vi "HFRR ADV v025 new software.vi"() -> ()   [LabVIEW 2025] (continued)
  # "Calibrates the ambient air temperature sensor. \nUsed for environmental chamber monitoring."
  # "Set B\n60 °C\nHigh-point calibration"
  # "Set A\n0 °C\nIce-point calibration"
  # "Set B\n60 °C\nHigh-point calibration"
  # "Set A\n0 °C\nIce-point calibration"
  # "Select Temperature Sensor"
  # "Choose which temperature sensor you are calibrating. Both use the same two-\npoint procedure: 0 °C (ice-point) and 60 °C (high-point)."
  # "Step 1 — Reference Instrument Setup"
  # "Connect a calibrated reference to the DUT port. This calibration performs two sets: one at 0 °C and one at 60 °C."
  # "Set A\n0 °C\nIce-point calibration"
  # "Set B\n60 °C\nHigh-point calibration"
  # "Allow the temperature bath to stabilise for at least 2 minutes at each set-point before recording the reading."
  # "Step 2 — Set A:  0 °C Calibration"
  # "Connect the  0 °C reference connector. Wait for the temperature to stabilise. Once stable, and click Record Point."
  # "Step 3 — Set A:  60 °C Calibration"
  # "Connect the  60 °C reference connector. Wait for the temperature to stabilise. Once stable, and click Record Point."
  # "Step 1 — Reference Instrument Setup"
  # "Connect a calibrated reference to the DUT port. This calibration performs two sets: one at 0 °C and one at 60 °C."
  # "Set A\n0 °C\nIce-point calibration"
  # "Set B\n60 °C\nHigh-point calibration"
  # "Allow the temperature bath to stabilise for at least 2 minutes at each set-point before recording the reading."
  # "Step 2 — Set A:  0 °C Calibration"
  # "Connect the  0 °C reference connector. Wait for the temperature to stabilise. Once stable, and click Record Point."
  # "Step 3 — Set A:  60 °C Calibration"
  # "Connect the  60 °C reference connector. Wait for the temperature to stabilise. Once stable, and click Record Point."
  # "System Control Commands\nS;1 - Starts the full automation cycle (Runs Priming-humidify till 70RH sequence first, then switches to Maintenance).\nS;0 - Stops the system immediately and enters Standby mode (Safe State: All actuators OFF).\nM;1 - Skips the priming sequence and jumps directly to Maintenance mode (PID control).\nR;1 - Resets the logic state machine and clears all errors, returning to Standby.\nService Mode (Manual Control)\nX;1 - Enters Manual Service Mode. This disables all automatic logic, sensor safety checks, and timers.\nX;0 - Exits Manual Service Mode and returns to Standby (Safe State).\nActuator Commands (Only work after sending X;1)\nP;[0-255] - Sets the Pump PWM. Note that this is Active Low (0 = Max Flow, 255 = Pump OFF).\nF;I;[0-255] - Sets the Intake Fan speed (0 = OFF, 255 = Max Speed).\nF;O;[0-255] - Sets the Exhaust Fan speed (0 = OFF, 255 = Max Speed).\nD;1 - Turns the Dehumidifier Relay ON.\nD;0 - Turns the Dehumidifier Relay OFF."
  # "%RH"
  # "ISO : WS1.4"
  # "Start test and end test log--- done\nDisable heater ON and Humidity ON during the test --- done\ntemprature and ---done\nhumidity reach log\nauto start run true logic and log\nmanual start log once"
  # "Reference Fluid Information"
  # "Note:\nMake sure to place all images in the folder \"C:\\WinDucom\\im\" before clicking on \"Import Image.\""
  # "NOTE:\nPlace all the images in the path \"C:\\WinDucom\\im\" before clicking on Import Image"
  # "Wear Scar Measurements"
  # "Reference Fluid Information"
  # "Graph :"
types:
  T1 = enum32{"Home", "Dashboard", "Imaging", "Report", "Analysis", "About", "Test Setup", "Advance", "Calibration"}
  T2 = enum32{"HOME", "Test Setup", "Acquire", "Adv Scar", "Adv Scar Report", "Compare Files", "Calibration", "About", "Advance", "Mooha"}
  T3 = enum16{"ASTM D6079", "ISO 12156", "CEC F-096-A-06", "Custom"}
  T4 = enum32{"Dashboard 1", "Dashboard 2", "Dashboard 3"}
  T5 = enum32{"COF", "Friction", "ECR", "Temperature", "Humidity", "Stroke"}
  T6 = enum32{"Coefficient Of Friction", "Air Temperature", "Humidity", "Stroke", "Sample Temperature", "Electrical Contact Resistance", "Frequency", "Air Temp vs Rh"}
  T7 = enum32{"Main", "Stroke", "Friction", "Temperature"}
  T8 = enum32{"Stroke Calibration", "Friction Force Calibration", "Temperature Calibration"}
  T9 = enum32{"Step 1", "Step 2", "Step 3", "Step 4", "Step 5", "Step 6", "Step 7", "Step 8", "Step 9"}
  T10 = enum32{"Test Progress", "Stroke Points Completed"}
  T11 = enum32{"Main", "Step 1", "Step 2", "Step 3", "Air Step 1", "Air Step 2", "Air Step 3"}
  T12 = enum32{"COMMUNICATION", "CALIBRATION", "Temp Variables", "Camera", "WO 2465 (1)", "WO 2465 (2)", "WO 2465 (3)"}
  T13 = typedef "Auto Start enum.ctl" = enum16{"Init", "Humidity & Temperature On", "Reach point", "Maintain Stage", "Start Stage", "close", "Exit"}
  T14 = typedef "imagedata.ctl" = cluster{"image type":i32, "image depth":i32, "image":u8[], "mask":u8[], "colors":u32[], "Rectangle":cluster{"left":i16, "top":i16, "right":i16, "bottom":i16}}
  T15 = enum32{"HOME", "Test Setup", "Acquire", "Compare Files", "Print Report", "About", "Advance", "Mooha"}
  T16 = cluster{"Read Heave and Surge":string, "Bytes at Heave Port":dbl, "Heave and Surge COM Port:":refnum<visa-resource-name>, "Com Port 2":refnum<visa-resource-name>, "Residual Due":string, "Heave COM Status 2":bool, "Heave COM Status":bool, "Port 2":bool, "Sway PPR":dbl, "Surge PPR":dbl, "Heave PPR":dbl, "Sway Pitch":dbl, "Surge Pitch":dbl, "Heave Pitch":dbl, "Sway Pulses/mm":dbl, "Surge Pulses/mm":dbl, "Heave Pulses/mm":dbl, "inner loop":dbl, "Read Heave and Surge 2":string, "String 36":string, "Write S":bool, "WriteCC1":string[], "Heave COM Loop":i32, "LastCom":string, "EXIT":bool, "Error Heave":errorcluster}
  T17 = enum8{"Enabled", "Disabled", "Disabled and Grayed Out"}
  T18 = enum32{"HOME", "Test Setup", "Acquire", "Adv Scar", "Adv Scar Report", "Compare Files", "About", "Advance", "Mooha"}
  T19 = typedef "POST ANALYSIS ENUM.ctl" = enum16{"OPEN EXE", "INIT", "OPEN FILE", "FIT", "DRAW REC", "DRAW LINE", "PAN", "ZOOM IN", "ZOOM OUT", "SET ZOOM", "CLEAR ROI", "GET MEASUREMENTS", "RESIZE MODE", "STREAM START", "STREAM STOP", "SHOW UI", "MINIMIZE UI", "HIDE UI", "CKISE APP", "CLOSE CONNECTION", "SAVE IMAGE", "SET ROI COLOR", "READ", "TCP CHECK", "CLOSE"}
  T20 = typedef "CAMERA LIVE FEED ENUM.ctl" = enum16{"OPEN EXE", "INIT", "READ", "CAMERA CONNECT", "CAMERA START", "CAMERA STOP", "CAMERA GRAY", "CAMERA RGB", "CAMERA MINIMIZE", "CAMERA CLOSE", "CAMERA MODE LIST", "CAMERA MODE SET", "CAMERA RESTORE", "CAMERA SAVE", "CLOSE"}
  T21 = enum16{"Always On", "Always Off", "Off While Running"}
  T22 = enum32{"Home", "Dashboard", "Imaging", "Report", "Analysis", "About", "Test Setup", "Advance"}
  T23 = cluster{"File Name":string, "Test Method":string, "Operator":string, "Fuel Description":string, "Date and time":string}
  T24 = enum32{"Home", "Dashboard", "Imaging", "Report", "Analysis", "About", "Test Setup"}
  T25 = enum32{"HOME", "Test Setup", "Acquire", "Compare Files", "About", "Advance", "Mooha"}
  T26 = enum16{"deny read/write", "deny write-only", "deny none"}
  T27 = typedef "NI_ReportGenerationCore.lvlib/HTML Report Image Alignment.ctl" = enum16{"(default)", "LEFT", "RIGHT", "TOP", "TEXTTOP", "MIDDLE", "ABSMIDDLE", "BASELINE", "BOTTOM", "ABSBOTTOM"}
  T28 = enum16{"open", "replace", "create", "open or create", "replace or create", "replace or create with confirmation"}
  T29 = enum16{"INIT", "READ", "MANUAL WRITE", "WRITE", "CLOSE", "ERROR INIT"}
  T30 = enum16{"open", "open or create", "create or replace", "create", "open (read only)"}
  T31 = cluster{"Mode":enum16{"RTU", "ASCII"}, "Slave Address":u8}
diagram:
  w3 = 0.0 ("ch0_filt")
  w5 = -9999999.0 ("max_ch0")
  w6 = 9999999.0 ("min_ch0")
  w17 = FALSE ("Visible")
  w18 = T17."Enabled" ("Disabled")
  w21 = FALSE ("Visible")
  w20 = FALSE ("Humidity Off Command")
  w36 = "" ("USER ID")
  (unwired) T18."HOME" ("Main Tab")
  # "[CH1]    - FF\n[CH2]   - TEMPERATURE\n[CH3]    - Humidity\n[CH4]    - AIR TEMP\n[CH5]\\- Visa Uno\n[CH6] \\- Visa Due\n[CH7]  \\- file path\n[CH8]   - Displacement Gain\n[CHA]   - Stroke Gain\n[CHB]   - Stroke PID Gain\n[CHC]   -Language Selection\n[CHD]   -Power +\n[CHE]   -Power_\n[CHF]   -Heater\n[CHG]   -Humidity Wet\n[CHH]   -Humidity Dry\n[CHI]   -Integral Time \n[CHIJ   -Air intercept\n[CHI]   -Temp Intercept"
  n1 = local write "Cal Password"("" ("Cal Password")) -> ()
  n2 = property on="Auto Start Test" class="Bool (strict)"("Visible"=TRUE) -> ()  [unwired: 2 in, 2 out]
  n3 = property on="FRICVALZ 2" class="Bool (strict)"("DisabledEnum"=w18) -> ()  [unwired: 2 in, 2 out]
  n4 = property on="FRICVALZ 4" class="Bool (strict)"("DisabledEnum"=w18) -> ()  [unwired: 2 in, 2 out]
  n5 = property on="FRICVALZ 3" class="Bool (strict)"("DisabledEnum"=w18) -> ()  [unwired: 2 in, 2 out]
  n6 = property on="About" class="Clust (strict)"("Visible"=FALSE) -> ()  [unwired: 2 in, 2 out]
  n7 = property on="Wrong Password" class="Str"("Visible"=w17) -> ()  [unwired: 2 in, 2 out]
  n8 = property on="Calibration 2" class="TabCtl (strict)"("Visible"=w17) -> ()  [unwired: 2 in, 2 out]
  n9 = flat-sequence {
    tunnel: [w58] -> w2
    tunnel: [w103] -> w28
    tunnel: w2 -> [w98]
    tunnel: [w104] -> w30
    tunnel: w28 -> [w104]
    tunnel: w30 -> [w167]
    tunnel: [w167] -> w29
    tunnel: w29 -> [w198]
    tunnel: [w198] -> w39
    tunnel: w39 -> [w205]
    tunnel: [w211] -> w27
    tunnel: [w199] -> w26
    tunnel: [w253] -> w1
    tunnel: [w252] -> _
    tunnel: w27 -> [w252]
    tunnel: w26 -> [w253]
    frame #0 {
      n10 = call "CLOSE CONNECTION.vi"("error in (no error)"="error in (no error) 2") -> ("error out"=w63:errorcluster)  [unwired: 10 in]
      n11 = call <vilib>:"Clear Errors.vi"("error in (no error)"=w63) -> ("error out"=w62:errorcluster)  [unwired: 5 in, 1 out]
      n12 = disable-structure shown="Enabled" {
        disable-tunnel: w62 -> [w90 _]
        disable-tunnel: [w89 _] -> w61
        frame Enabled {
          n13 = call <userlib>:"Fit VI window to Largest Dec.vi"("error in (no error)"=w90, "border spacing (2 px)"=1) -> ("error out"=w93:errorcluster, "dup VI Ref"=w97:refnum<vi>)  [unwired: 4 in]
          n14 = invoke on="Invoke Node" class="VI" method="FP.Run-Time Position.Maximized"(reference=w97, error in=w93) -> (error out=w94:errorcluster)  [unwired: 2 in, 3 out]
          n15 = call <vilib>:"Clear Errors.vi"("error in (no error)"=w94) -> ("error out"=w96:errorcluster)  [unwired: 5 in, 1 out]
          n16 = control-ref of="This VI"() -> (w88:refnum<vi>)
          n17 = invoke on="Invoke Node" class="VI" method="Default Vals.Reinit All"(reference=w88, error in=w96) -> (reference out=w92:refnum<vi>, error out=w91:errorcluster)  [unwired: 1 in, 1 out]
          n18 = Close Reference(reference=w92, error in (no error)=w91) -> (error out=w89:errorcluster)
        }
        frame Disabled {
        }
      }
      n19 = call "Stall Data Flow.vim"("value in"=w61, "milliseconds to wait"=u32 2000) -> ("value out"=w60:errorcluster)  [unwired: 1 out]
      n20 = call "Read Config.vi"("error in (no error)"=w60) -> ("error out"=w58:errorcluster, "STROKE PARAMETERS"=w69:dbl[], "ADC PARAMETERS"=w70:dbl[], "PID  PARAMETERS"=w71:dbl[], "Stroke Calibration"=w68:string)  [unwired: 6 in]
      n21 = Index Array(array=w69) -> (element #1=w86:dbl, element #2=w87:dbl)  [unwired: 2 in]
      n22 = Index Array(array=w70) -> (element #1=w82:dbl, element #2=w83:dbl, element #3=w84:dbl, element #4=w85:dbl)  [unwired: 4 in]
      n23 = Index Array(array=w71) -> (element #1=w73:dbl, element #2=w74:dbl, element #3=w75:dbl, element #4=w76:dbl, element #5=w77:dbl, element #6=w78:dbl, element #7=w79:dbl, element #8=w80:dbl, element #9=w81:dbl)  [unwired: 9 in]
      n24 = local write "milliseconds to wait"(w73) -> ()
      n25 = local write "dt"(w74) -> ()
      n26 = local write "kp"(w75) -> ()
      n27 = local write "ki"(w76) -> ()
      n28 = local write "kd"(w77) -> ()
      n29 = local write "max_step_change"(w78) -> ()
      n30 = local write "max_amplitude"(w79) -> ()
      n31 = local write "min_amplitude"(w80) -> ()
      n32 = local write "startup_cmd"(w81) -> ()
      n33 = local write "VREF"(w82) -> ()
      n34 = local write "ADC_Resolution"(w83) -> ()
      n35 = local write "PIEZO_CAL_FACTOR"(w84) -> ()
      n36 = local write "NORMAL_FORCE"(w85) -> ()
      n37 = local write "STROKE FILTER"(w86) -> ()
      n38 = local write "Add up Stroke"(w87) -> ()
      n39 = Spreadsheet String To Array(delimiter (Tab)=";", format string="", spreadsheet string=w68, array type (2D Dbl)=dbl[] []) -> (array=w72:dbl[])
      n40 = local write "calibration values"(w72) -> ()
    }
    frame #1 {
      n41 = property on="Auto Scar Check" class="Clust (strict)"("Visible"=TRUE) -> ()  [unwired: 2 in, 2 out]
      n42 = property on="Sign In" class="Bool (strict)"("DisabledEnum"=T17."Disabled" ("Disabled")) -> ()  [unwired: 2 in, 2 out]
      n43 = local write "sign in temp"(FALSE ("sign in temp")) -> ()
      n44 = call "dialog box.vi"("Status"="Before starting the test, verify that the microscope cable is connected.", "error in"=w98) -> ("error out"=w103:errorcluster)  [unwired: 8 in]
    }
    frame #2 {
      (unwired) TRUE ("Re-Initialise")
      w110 = FALSE ("Upld AR 2")
      # "kkkkk"
      # "C:\\Windows\\wndcm_pw_stdED hfrr.txt"
      # "C:\\LAB-IQ NXT"
      # "C:\\LAB-IQ NXT\\wndcm_pw_stdED hfrr.txt"
      # "password file"
      n45 = Current VI's Path() -> (path=w123:path)
      n46 = Strip Path(path=w123) -> (stripped path=w116:path)  [unwired: 1 out]
      n47 = local write "Json End Flg"(w110) -> ()
      n48 = local write "Json St Flg"(w110) -> ()
      n49 = local write "main tab sub"(enum32{"Page 1", "Page 2"}."Page 1" ("main tab sub")) -> ()
      n50 = local write "Main Tab Display"(T4."Dashboard 1" ("Main Tab Display")) -> ()
      n51 = local write "Main Tab"(T2."HOME" ("Main Tab")) -> ()
      n52 = Path To String(path=w116) -> (string=w118:string)
      n53 = Search/Split String(string=w118, search string/char (-)=".exe") -> (match + rest of string=w120:string)  [unwired: 1 in, 2 out]
      n54 = Match True/False String(2:".vi" ("false string"), 3:".exe" ("true string"), 4:w120) -> (0:w117:bool)  [unwired: 1 out]
      n55 = List Folder(path=path "C:/LAB-IQ" ("directory path"), pattern="*.txt") -> (filenames=w129:string[])  [unwired: 2 in, 3 out]
      n56 = case shown="True" w117 {
        tunnel: w116 -> [w138 w140]
        tunnel: [w138 w139] -> w114
        frame False {
        }
        frame True {
          n57 = Strip Path(path=w140) -> (stripped path=w139:path)  [unwired: 1 out]
        }
      }
      n58 = Search 1D Array(1D array=w129, element="wndcm_pw_stdED hfrr.txt") -> (index of element=w132:i32)  [unwired: 1 in]
      n59 = Equal?(x=w132, y=-1) -> (x = y?=w127:bool)
      n60 = Path To String(path=w114) -> (string=→"Gain path":string)
      n61 = case shown="True" w127 {
        frame False {
        }
        frame True {
          n62 = String To Byte Array(string="123\n") -> (unsigned byte array=w145:u8[])
          n63 = Array Size(array=w145) -> (size(s)=w144:i32)
          n64 = for {
            N: w144 -> [_]
            tunnel: w145 -> [w158]
            tunnel: [w155] -> w147 mode=indexing
            tunnel: w144 -> [w150]
            i -> [w148]
            n65 = Decrement(x=w150) -> (x-1=w151:i32)
            n66 = Index Array(array=w158, index=w148) -> (element=w157:u8)
            n67 = Equal?(x=w148, y=w151) -> (x = y?=w152:bool)
            n68 = Number To Decimal String(number=w157) -> (decimal integer string=w156:string)  [unwired: 1 in]
            n69 = Select(t="", s=w152, f="\r") -> (s? t:f=w149:string)
            n70 = Concatenate Strings(w156, w149) -> (w155:string)
          }
          n71 = local read "file path"() -> (w141:path)
          n72 = Concatenate Strings(w147) -> (w143:string)
          n73 = call <vilib>:"Write Characters To File.vi"("append to file? (new file:F)"=FALSE, "character string"=w143, "file path (dialog if empty)"=w141) -> ()  [unwired: 2 in, 1 out]
        }
      }
      n74 = local write "FLAG 2"(0.0 ("FLAG 2")) -> ()
      n75 = local write "conststatus"(0.0 ("rpm value : 2")) -> ()
      n76 = local write "EVENT LOG"("") -> ()
      n77 = local write "COUNT"(0 ("COUNT")) -> ()
      n78 = local write "clk"(0.0 ("clk")) -> ()
      n79 = local write "Flag"(0.0 ("Flag")) -> ()
      n80 = local write "Lan flag"(0.0 ("Lan flag")) -> ()
      n81 = local write "Com flag"(u32 0 ("Com flag")) -> ()
      n82 = local write "refresh flag"(FALSE ("refresh flag")) -> ()
      n83 = local write "Upld AR 2"(TRUE ("Upld AR 2")) -> ()
      "file path" <- path "C:/LAB-IQ/wndcm_pw_stdED hfrr.txt" ("file path")
      "FF buffer" <- dbl[] [] ("FF buffer")
    }
    frame #3 {
      # "C:\\WinDucom\\calibrate WO 2391.dcf"
      n84 = String To Path(string="C:\\LAB-IQ\\Image Calibrate v01.dcf") -> (path=w162:path)
      n85 = String To Path(string="C:\\LAB-IQ\\calibrate WO 2465.dcf") -> (path=w166:path)
      n86 = Open/Create/Replace File "Open File"(file path (use dialog)=w166) -> (refnum out=w165:refnum<file>)  [unwired: 5 in, 2 out]
      n87 = Open/Create/Replace File ("Open File")(file path (use dialog)=w162) -> (refnum out=w161:refnum<file>)  [unwired: 5 in, 2 out]
      n88 = for {
        N: 4 -> [_]
        tunnel: w161 -> [w173]
        i -> [w169]
        n89 = Read from Text File ("Read File")(file (use dialog)=w173) -> (text=w174:string)  [unwired: 3 in, 3 out]
        n90 = String Subset(string=w174, offset (0)=6, length (rest)=10 ("length (rest)")) -> (substring=w170:string)
        n91 = Fract/Exp String To Number(string=w170) -> (number=w168:dbl)  [unwired: 3 in, 1 out]
        n92 = case shown="3" w169 {
          tunnel: w168 -> [w175 w176 _ w177 _]
          frame 0 {
            n93 = local write "5x Gain"(w175) -> ()
          }
          frame 1 {
            n94 = local write "10x Gain"(w176) -> ()
          }
          frame 2 {
          }
          frame 3 {
            n95 = local write "100x gain"(w177) -> ()
          }
          frame 4, Default {
          }
        }
      }
      n96 = for {
        N: 24 -> [_]
        tunnel: w165 -> [w186]
        i -> [w180]
        (unwired) TRUE ("line mode (F)")
        n97 = Read from Text File "Read File"(file (use dialog)=w186) -> (text=w185:string)  [unwired: 3 in, 3 out]
        n98 = Match Pattern(string=w185, regular expression="]") -> (after substring=w183:string)  [unwired: 1 in, 3 out]
        n99 = String Subset(string=w185, offset (0)=5, length (rest)=10 ("length (rest)")) -> (substring=w178:string)
        n100 = Fract/Exp String To Number(string=w178) -> (number=w179:dbl)  [unwired: 3 in, 1 out]
        n101 = Match Pattern(string=w183, regular expression="-") -> (before substring=w181:string)  [unwired: 1 in, 3 out]
        n102 = case shown="18" w180 {
          tunnel: w179 -> [_ _ _ _ _ _ _ _ _ _ w193 _ _ _ _ _ _ _ _ _ _ _ _ _ _]
          tunnel: w181 -> [_ _ _ _ w189 w190 w191 _ _ _ _ _ _ _ _ _ _ _ _ _ w194 _ w195 w196 _]
          frame 0 {
          }
          frame 1 {
          }
          frame 2 {
          }
          frame 3 {
          }
          frame 4 {
            n103 = local write "Com Port 1"(w189) -> ()
          }
          frame 5 {
            n104 = local write "Com Port 2"(w190) -> ()
            n105 = local write "visa due"(w190) -> ()
          }
          frame 6 {
            n106 = String To Path(string=w191) -> (path=w192:path)
            n107 = local write "File Path"(w192) -> ()
          }
          frame 7 {
          }
          frame 8 {
          }
          frame 9 {
          }
          frame 10 {
            n108 = local write "Language Selection"(w193) -> ()
          }
          frame 11 {
          }
          frame 12 {
          }
          frame 13 {
          }
          frame 14 {
          }
          frame 15 {
          }
          frame 16 {
          }
          frame 17 {
          }
          frame 18 {
          }
          frame 21 {
          }
          frame 22 {
            n109 = local write "Com Port 3"(w194) -> ()
          }
          frame 23 {
          }
          frame 19 {
            n110 = local write "C3 :"(w195) -> ()
          }
          frame 20 {
            n111 = local write "Camera Port :"(w196) -> ()
          }
          frame 24, Default {
          }
        }
      }
    }
    frame #4 {
      n112 = Wait (ms)(milliseconds to wait=u32 1000) -> ()  [unwired: 1 out]
    }
    frame #5 {
      w214 = u32 2000 ("milliseconds to wait")
      w241 = u32 2000 ("milliseconds to wait")
      n113 = call "CAMERA LIVE FEED FGV.vi"("Enum - Menu"=CAMERA_LIVE_FEED_ENUM."OPEN EXE", "error in (no error)"=w205) -> ("error out"=w247:errorcluster)  [unwired: 8 in, 1 out]
      n114 = call "IMAGE ANALYSIS.vi"("Enum"=POST_ANALYSIS_ENUM."OPEN EXE", "error in"=w205) -> ("error out"=w202:errorcluster)  [unwired: 8 in, 1 out]
      n115 = call "Stall Data Flow.vim"("value in"=w247, "milliseconds to wait"=w241) -> ("value out"=w245:errorcluster)  [unwired: 1 out]
      n116 = call "Stall Data Flow.vim"("value in"=w202, "milliseconds to wait"=u32 8000) -> ("value out"=w201:errorcluster)  [unwired: 1 out]
      n117 = call "CAMERA LIVE FEED FGV.vi"("Enum - Menu"=CAMERA_LIVE_FEED_ENUM."INIT", "error in (no error)"=w245) -> ("error out"=w243:errorcluster)  [unwired: 8 in, 1 out]
      n118 = call "IMAGE ANALYSIS.vi"("Enum"=POST_ANALYSIS_ENUM."INIT", "error in"=w201) -> ("error out"=w199:errorcluster)  [unwired: 8 in, 1 out]
      n119 = case shown="Error .." w243 {
        selector: w243 -> [w248 _]
        tunnel: [w248 _] -> w242
        frame No Error {
        }
        frame Error {
          n120 = One Button Dialog(message="Camera initialization error.\nPlease Restart the software") -> ()  [unwired: 1 in, 1 out]
        }
      }
      n121 = property on="Camera Port :" class="CmbBox"() -> ("Strings[]"=w239:string[], "Value"=w240:string)  [unwired: 2 in, 2 out]
      n122 = Search 1D Array(1D array=w239, element=w240) -> (index of element=w238:i32)  [unwired: 1 in]
      n123 = Type Cast(type=30, x=w238) -> (*(type *) &x=w236:i32)
      n124 = call "Stall Data Flow.vim"("value in"=w242, "milliseconds to wait"=w241) -> ("value out"=w218:errorcluster)  [unwired: 1 out]
      n125 = Add(x=w236, y=48) -> (x+y=w217:i32)
      n126 = call "CAMERA LIVE FEED FGV.vi"("Enum - Menu"=CAMERA_LIVE_FEED_ENUM."CAMERA CONNECT", "error in (no error)"=w218, "CAMERA PORT"=w217) -> ("error out"=w227:errorcluster)  [unwired: 7 in, 1 out]
      n127 = call "Stall Data Flow.vim"("value in"=w227, "milliseconds to wait"=u32 5000) -> ("value out"=w228:errorcluster)  [unwired: 1 out]
      n128 = call "CAMERA LIVE FEED FGV.vi"("Enum - Menu"=CAMERA_LIVE_FEED_ENUM."CAMERA MODE LIST", "error in (no error)"=w228) -> ("error out"=w230:errorcluster)  [unwired: 8 in, 1 out]
      n129 = call "Stall Data Flow.vim"("value in"=w230, "milliseconds to wait"=w214) -> ("value out"=w229:errorcluster)  [unwired: 1 out]
      n130 = call "CAMERA LIVE FEED FGV.vi"("Enum - Menu"=CAMERA_LIVE_FEED_ENUM."READ", "error in (no error)"=w229) -> ("error out"=w216:errorcluster, "data out"=→"Camera List":string)  [unwired: 8 in]
      n131 = Type Cast(type=30, x=0) -> (*(type *) &x=w210:i32)
      n132 = call "Stall Data Flow.vim"("value in"=w216, "milliseconds to wait"=w214) -> ("value out"=w215:errorcluster)  [unwired: 1 out]
      n133 = Add(x=w210, y=48) -> (x+y=w208:i32)
      n134 = call "CAMERA LIVE FEED FGV.vi"("Enum - Menu"=CAMERA_LIVE_FEED_ENUM."CAMERA MODE SET", "error in (no error)"=w215, "CAMERA MODE"=w208) -> ("error out"=w212:errorcluster)  [unwired: 7 in, 1 out]
      n135 = call "Stall Data Flow.vim"("value in"=w212, "milliseconds to wait"=u32 2000) -> ("value out"=w232:errorcluster)  [unwired: 1 out]
      n136 = call "CAMERA LIVE FEED FGV.vi"("Enum - Menu"=CAMERA_LIVE_FEED_ENUM."CAMERA START", "error in (no error)"=w232) -> ("error out"=w233:errorcluster)  [unwired: 8 in, 1 out]
      n137 = call "Stall Data Flow.vim"("value in"=w233, "milliseconds to wait"=u32 1000) -> ("value out"=w234:errorcluster)  [unwired: 1 out]
      n138 = call "CAMERA LIVE FEED FGV.vi"("Enum - Menu"=CAMERA_LIVE_FEED_ENUM."CAMERA MINIMIZE", "error in (no error)"=w234) -> ("error out"=w211:errorcluster)  [unwired: 8 in, 1 out]
    }
    frame #6 {
      n139 = case shown="No Error" w252 {
        frame No Error {
          n140 = property on="Auto Scar Check" class="Clust (strict)"("Visible"=FALSE) -> ()  [unwired: 2 in, 2 out]
        }
        frame Error {
        }
      }
      n141 = property on="Sign In" class="Bool (strict)"("DisabledEnum"=T17."Enabled" ("Disabled")) -> ()  [unwired: 2 in, 2 out]
      n142 = local write "sign in temp"(TRUE ("sign in temp")) -> ()
    }
  }
  n143 = local write "SCAR MEASURMENT"(enum32{"Auto Scar", "Manual Scar"}."Manual Scar" ("SCAR MEASURMENT")) -> ()
  n144 = local write "Temperature Off Command"(w20) -> ()
  n145 = local write "Main Dashboard Buttons"(T1."Home" ("Main Dashboard Buttons")) -> ()
  n146 = local write "Humidity Off Command"(w20) -> ()
  n147 = local write "CAMERA ROI MIN TEMP"(w20) -> ()
  n148 = local write "TEST FILE NAM,E SAVED"(w20) -> ()
  n149 = local write "LIVE FEED MIN TEMP"(w20) -> ()
  n150 = local write "SCAR MEASURMENT"(enum32{"Auto Scar", "Manual Scar"}."Manual Scar" ("SCAR MEASURMENT")) -> ()
  n151 = local write "Auto stop temp"(w21) -> ()
  n152 = local write "main tab sub"(enum32{"Page 1", "Page 2"}."Page 1" ("main tab sub")) -> ()
  n153 = local write "USERNAME"(w36) -> ()
  n154 = local write "Main Tab"(T2."HOME" ("Main Tab")) -> ()
  n155 = local write "USER ID"(w36) -> ()
  n156 = property on="Auto Scar Check  2" class="Clust (strict)"("Visible"=w21) -> (error out=w24:errorcluster)  [unwired: 2 in, 1 out]
  n157 = property on="Quit" class="Bool (strict)"("Value"=FALSE ("Quit")) -> (error out=w38:errorcluster)  [unwired: 2 in, 1 out]
  n158 = while {
    stop <- w255 stop-if-true
    n159 = event shown="[12] \"Cal Password\": Value Change" {
      selector: _ -> [_ _ _ _ _ _ _ _ _ _ _ _ _ _ _ _ _ _ _ _ _ _ _ _ _ _ _ _ _ _ _ _ _ _ _ _ _ _ _]
      dyn-events: _ -> [_ _ _ _ _ _ _ _ _ _ _ _ _ _ _ _ _ _ _ _ _ _ _ _ _ _ _ _ _ _ _ _ _ _ _ _ _ _ _]
      timeout: 100 -> [_ _ _ _ _ _ _ _ _ _ _ _ _ _ _ _ _ _ _ _ _ _ _ _ _ _ _ _ _ _ _ _ _ _ _ _ _ _ _]
      tunnel: [FALSE FALSE _ FALSE _ _ _ _ _ _ _ _ _ _ _ _ _ _ _ _ _ _ _ _ _ _ _ _ _ _ _ _ _ _ _ _ _ _ TRUE] -> w255
      event Timeout {
        n160 = event-data() -> ()  [unwired: 1 in, 3 out]
        n161 = disable-structure shown="Disabled" {
          frame Disabled {
            n162 = local read "Auto Start Test"() -> (w269:bool)
            n163 = local read "RUN"() -> (w270:bool)
            n164 = Or(x=w270, y=w269) -> (x .or. y?=w268:bool)
            n165 = case shown="True" w268 {
              frame False {
                w271 = TRUE ("PAUSE")
                n166 = call "ELAPSED TIMER VI - abort test.vi"("RESET"=w271, "PAUSE"=w271) -> ()  [unwired: 7 in, 3 out]
              }
              frame True {
                n167 = local read "Stroke 2"() -> (w276:dbl)
                n168 = local read "FF 3"() -> (w278:dbl)
                n169 = Equal?(x=w276, y=0.95 ("Stroke 2")) -> (x = y?=w273:bool)
                n170 = Equal?(x=w278, y=0.0 ("FF 3")) -> (x = y?=w274:bool)
                n171 = Or(x=w274, y=w273) -> (x .or. y?=w272:bool)
                n172 = case shown="True" w272 {
                  selector: w272 -> [_ w283]
                  frame False {
                    w279 = TRUE ("PAUSE")
                    n173 = call "ELAPSED TIMER VI - abort test.vi"("RESET"=w279, "PAUSE"=w279) -> ()  [unwired: 7 in, 3 out]
                  }
                  frame True {
                    n174 = Not(x=w283) -> (.not. x?=w282:bool)
                    n175 = call "ELAPSED TIMER VI - abort test.vi"("TARGET"=60.0, "RESET"=w282, "PAUSE"=FALSE) -> ("ELAPSED INDICATION"=w280:bool)  [unwired: 6 in, 2 out]
                    n176 = case shown="True" w280 {
                      frame False {
                      }
                      frame True {
                        n177 = stacked-sequence {
                          frame #0 {
                            w285 = FALSE
                            n178 = local write "RUN"(w285) -> ()
                            n179 = local write "Auto Start Test"(w285) -> ()
                          }
                          frame #1 {
                            n180 = One Button Dialog(message="Test stopped due to a communication error. Reconnect the C1 and C2 cables.") -> ()  [unwired: 1 in, 1 out]
                          }
                        }
                      }
                    }
                  }
                }
              }
            }
          }
          frame Enabled {
          }
        }
        n181 = Get Date/Time In Seconds() -> (seconds since 1Jan1904=w266:timestamp)
        n182 = Format Into String(format string="%<%I:%M:%S:%p %d:%B:%Y>T", w266) -> (resulting string=→"Time Stamp":string)  [unwired: 2 in, 1 out]
        n183 = local read "Service Password enable"() -> (w258:bool)
        n184 = local read "FILE"() -> (w263:string)
        n185 = call <vilib>:"Trim Whitespace.vi"("string"=w263) -> ("trimmed string"=w262:string)  [unwired: 1 in]
        n186 = String Length(string=w262) -> (length=w261:i32)
        n187 = Greater?(x=w261, y=1) -> (0:w259:bool)
        n188 = case shown="False" w259 {
          tunnel: w258 -> [w287 _]
          frame False {
            n189 = case shown="False" w287 {
              frame True {
                w288 = "Test Start In Service Mode" ("Tip Strip")
                w289 = T17."Enabled" ("Disabled")
                n190 = property on="Auto Start Test" class="Bool (strict)"("DisabledEnum"=w289, "TipStrip"=w288) -> ()  [unwired: 2 in, 2 out]
                n191 = property on="RUN" class="Bool (strict)"("DisabledEnum"=w289, "TipStrip"=w288) -> ()  [unwired: 2 in, 2 out]
              }
              frame False {
                w290 = "Enter File Name to Start Test" ("Tip Strip")
                w291 = T17."Disabled and Grayed Out" ("Disabled")
                n192 = property on="Auto Start Test" class="Bool (strict)"("DisabledEnum"=w291, "TipStrip"=w290) -> ()  [unwired: 2 in, 2 out]
                n193 = property on="RUN" class="Bool (strict)"("DisabledEnum"=w291, "TipStrip"=w290) -> ()  [unwired: 2 in, 2 out]
              }
            }
          }
          frame True {
            w292 = "" ("Tip Strip")
            w293 = T17."Enabled" ("Disabled")
            n194 = property on="Auto Start Test" class="Bool (strict)"("DisabledEnum"=w293, "TipStrip"=w292) -> ()  [unwired: 2 in, 2 out]
            n195 = property on="RUN" class="Bool (strict)"("DisabledEnum"=w293, "TipStrip"=w292) -> ()  [unwired: 2 in, 2 out]
          }
        }
      }
      event "RUN": Value Change {
        n196 = event-data() -> ()  [unwired: 1 in, 6 out]
        n197 = local read "RUN"() -> (w295:bool)
        n198 = case shown="False" w295 {
          frame False {
            n199 = flat-sequence {
              frame #0 {
                n200 = local write "START TEMP"(FALSE ("START TEMP")) -> ()
              }
              frame #1 {
                n201 = Wait (ms)(milliseconds to wait=u32 1500) -> ()  [unwired: 1 out]
              }
              frame #2 {
              }
              frame #3 {
                n202 = local write "Due Write"("VC;0") -> ()
              }
              frame #4 {
                n203 = Wait (ms)(milliseconds to wait=u32 1500) -> ()  [unwired: 1 out]
              }
              frame #5 {
                w304 = T17."Enabled" ("Disabled")
                (unwired) T22."Imaging" ("Main Dashboard Buttons")
                (unwired) T18."Adv Scar" ("Main Tab")
                w306 = "" ("FILE")
                n204 = local write "measured_stroke"(0.0 ("measured_stroke")) -> ()
                n205 = local write "Due Write"("VC;0") -> ()
                n206 = local write "FILE"(w306) -> ()
                n207 = local write "Batch Ref Num :"(w306) -> ()
                n208 = local write "Fuel Discription :"(w306) -> ()
                n209 = local write "Main Tab"(T2."Adv Scar" ("Main Tab")) -> ()
                n210 = local write "Remarks :"(w306) -> ()
                n211 = local write "Main Dashboard Buttons"(T1."Imaging" ("Main Dashboard Buttons")) -> ()
                n212 = local write "TEST FILE NAM,E SAVED"(FALSE ("TEST FILE NAM,E SAVED")) -> ()
                n213 = property on="Stroke ( mm )" class="WFChart (strict)"("History Data"=cluster{"y":dbl, dbl, "y":dbl}[] []) -> ()  [unwired: 2 in, 2 out]
                n214 = property on="Auto Start Test" class="Bool (strict)"("Visible"=TRUE) -> ()  [unwired: 2 in, 2 out]
                n215 = property on="FRICVALZ 2" class="Bool (strict)"("DisabledEnum"=w304) -> ()  [unwired: 2 in, 2 out]
                n216 = property on="FRICVALZ 4" class="Bool (strict)"("DisabledEnum"=w304) -> ()  [unwired: 2 in, 2 out]
                n217 = property on="FRICVALZ 3" class="Bool (strict)"("DisabledEnum"=w304) -> ()  [unwired: 2 in, 2 out]
              }
            }
          }
          frame True {
            n218 = flat-sequence {
              frame #0 {
                n219 = local write "Due Write"("VC;1") -> ()
              }
              frame #1 {
                n220 = Wait (ms)(milliseconds to wait=u32 2000) -> ()  [unwired: 1 out]
              }
              frame #2 {
                n221 = local write "Due Write"("VC;1") -> ()
              }
              frame #3 {
                n222 = Wait (ms)(milliseconds to wait=u32 2000) -> ()  [unwired: 1 out]
              }
              frame #4 {
                w314 = T17."Disabled" ("Disabled")
                n223 = property on="Auto Start Test" class="Bool (strict)"("Visible"=FALSE) -> ()  [unwired: 2 in, 2 out]
                n224 = local write "START TEMP"(TRUE ("START TEMP")) -> ()
                n225 = property on="FRICVALZ 2" class="Bool (strict)"("DisabledEnum"=w314) -> ()  [unwired: 2 in, 2 out]
                n226 = property on="FRICVALZ 4" class="Bool (strict)"("DisabledEnum"=w314) -> ()  [unwired: 2 in, 2 out]
                n227 = property on="FRICVALZ 3" class="Bool (strict)"("DisabledEnum"=w314) -> ()  [unwired: 2 in, 2 out]
              }
            }
          }
        }
      }
      event "Auto": Value Change {
        n228 = event-data() -> ()  [unwired: 1 in, 6 out]
        n229 = stacked-sequence {
          frame #0 {
            n230 = local write "FILE"("") -> ()
          }
          frame #1 {
            n231 = Get Date/Time In Seconds() -> (seconds since 1Jan1904=w320:timestamp)
            n232 = Format Into String(format string="%<%I_%M_%S_%p_%d_%B_%Y>T", w320) -> (resulting string=w319:string)  [unwired: 2 in, 1 out]
            n233 = local write "FILE"(w319) -> ()
          }
        }
        n234 = local read "Auto"() -> (w317:bool)
        n235 = Not(x=w317) -> (.not. x?=w316:bool)
        n236 = local write "Auto"(w316) -> ()
      }
      event "Auto Start Temp": Value Change {
        n237 = event-data() -> ()  [unwired: 1 in, 6 out]
        n238 = local read "Auto Start Test"() -> (w323:bool)
        n239 = case shown="False" w323 {
          frame False {
            n240 = stacked-sequence {
              frame #0 {
                n241 = local write "START TEMP"(FALSE ("START TEMP")) -> ()
              }
              frame #1 {
                n242 = Wait (ms)(milliseconds to wait=u32 2000) -> ()  [unwired: 1 out]
              }
              frame #2 {
                n243 = local write "Due Write"("VC;0") -> ()
              }
              frame #3 {
                n244 = Wait (ms)(milliseconds to wait=u32 2000) -> ()  [unwired: 1 out]
              }
              frame #4 {
                w333 = T17."Enabled" ("Disabled")
                (unwired) T22."Imaging" ("Main Dashboard Buttons")
                w334 = "" ("FILE")
                n245 = local write "Main Tab"(T2."Adv Scar" ("Main Tab")) -> ()
                n246 = local write "measured_stroke"(0.0 ("measured_stroke")) -> ()
                n247 = local write "Main Dashboard Buttons"(T1."Imaging" ("Main Dashboard Buttons")) -> ()
                n248 = property on="RUN" class="Bool (strict)"("Visible"=TRUE) -> ()  [unwired: 2 in, 2 out]
                n249 = local write "Due Write"("VC;0") -> ()
                n250 = local write "TEST FILE NAM,E SAVED"(FALSE ("TEST FILE NAM,E SAVED")) -> ()
                n251 = local write "Fuel Discription :"(w334) -> ()
                n252 = local write "Batch Ref Num :"(w334) -> ()
                n253 = local write "Remarks :"(w334) -> ()
                n254 = local write "FILE"(w334) -> ()
                n255 = property on="FRICVALZ 2" class="Bool (strict)"("DisabledEnum"=w333) -> ()  [unwired: 2 in, 2 out]
                n256 = property on="FRICVALZ 4" class="Bool (strict)"("DisabledEnum"=w333) -> ()  [unwired: 2 in, 2 out]
                n257 = property on="FRICVALZ 3" class="Bool (strict)"("DisabledEnum"=w333) -> ()  [unwired: 2 in, 2 out]
              }
            }
          }
          frame True {
            n258 = flat-sequence {
              frame #0 {
                n259 = local write "Due Write"("VC;1") -> ()
              }
              frame #1 {
                n260 = Wait (ms)(milliseconds to wait=u32 2000) -> ()  [unwired: 1 out]
              }
              frame #2 {
                n261 = local write "Due Write"("VC;1") -> ()
              }
              frame #3 {
                n262 = Wait (ms)(milliseconds to wait=u32 2000) -> ()  [unwired: 1 out]
              }
              frame #4 {
                w341 = T17."Disabled" ("Disabled")
                n263 = property on="RUN" class="Bool (strict)"("Visible"=FALSE) -> ()  [unwired: 2 in, 2 out]
                n264 = property on="FRICVALZ 2" class="Bool (strict)"("DisabledEnum"=w341) -> ()  [unwired: 2 in, 2 out]
                n265 = property on="FRICVALZ 4" class="Bool (strict)"("DisabledEnum"=w341) -> ()  [unwired: 2 in, 2 out]
                n266 = property on="FRICVALZ 3" class="Bool (strict)"("DisabledEnum"=w341) -> ()  [unwired: 2 in, 2 out]
                "START TEMP" <- TRUE
              }
            }
          }
        }
      }
      event "FILE", "USERNAME", "USER ID": Mouse Enter {
        n267 = event-data() -> ()  [unwired: 1 in, 4 out]
        n268 = dll-call lib="kernel32.dll" fn="Wow64DisableWow64FsRedirection"("OldValue"=0) -> (error out=w348:errorcluster, "OldValue"=w346:i32)  [unwired: 4 in, 1 out]
        n269 = call <vilib>:"System Exec.vi"("run minimized? (F)"=TRUE, "error in (no error)"=w348, "command line"="C:\\Program Files\\Common Files\\Microsoft Shared\\Ink\\TabTip.exe") -> ("error out"=w347:errorcluster)  [unwired: 5 in, 3 out]
        n270 = dll-call lib="kernel32.dll" fn="Wow64EnableWow64FsRedirection"(error in=w347, "OldValue"=w346) -> ()  [unwired: 4 in, 2 out]
      }
      event "EDIT": Value Change {
        n271 = event-data() -> ()  [unwired: 1 in, 6 out]
        n272 = local read "EDIT"() -> (w349:bool)
        n273 = case shown="False" w349 {
          frame False {
            n274 = control-ref of="This VI"() -> (w366:refnum<vi>)
            n275 = property class="VI"(reference=w366) -> (reference out=w357:refnum<vi>, error out=w361:errorcluster, "Panel"=w365:refnum<vi>)  [unwired: 1 in]
            n276 = property class="Pnl"(reference=w365, error in=w361) -> (reference out=w359:refnum<vi>, error out=w362:errorcluster, "Panes[]"=w364:refnum<vi>[])
            n277 = for {
              tunnel: w364 -> [w372] mode=indexing
              tunnel: T21."Always Off" ("Horizontal Scrollbar Visibility") -> [w371]
              tunnel: w362 -> [w368]
              tunnel: [w367] -> w360
              n278 = property class="Pane"(reference=w372, error in=w368, "HorizScrollbarVisibility"=w371) -> (reference out=w369:refnum<vi>, error out=w370:errorcluster)
              n279 = Close Reference(reference=w369, error in (no error)=w370) -> (error out=w367:errorcluster)
            }
            n280 = Close Reference(reference=w359, error in (no error)=w360) -> (error out=w358:errorcluster)
            n281 = Close Reference(reference=w357, error in (no error)=w358) -> (error out=w352:errorcluster)
            "error out 7" <- w352
            n282 = call <vilib>:"Clear Errors.vi"("error in (no error)"=w352) -> ("error out"=w351:errorcluster)  [unwired: 5 in, 1 out]
            n283 = local write "Service Password enable"(FALSE ("Service Password enable")) -> ()
            n284 = call <userlib>:"Fit VI window to Largest Dec.vi"("error in (no error)"=w351, "border spacing (2 px)"=1) -> ("error out"=w356:errorcluster, "dup VI Ref"=w354:refnum<vi>)  [unwired: 4 in]
            n285 = invoke on="Invoke Node" class="VI" method="FP.Run-Time Position.Maximized"(reference=w354, error in=w356) -> (error out=w355:errorcluster)  [unwired: 2 in, 3 out]
            n286 = call <vilib>:"Clear Errors.vi"("error in (no error)"=w355) -> ()  [unwired: 5 in, 2 out]
          }
          frame True {
          }
        }
      }
      event "Heater Button": Value Change {
        n287 = event-data() -> ()  [unwired: 1 in, 6 out]
        n288 = local read "Heater Button"() -> (w373:bool)
        n289 = case shown="True" w373 {
          frame True {
            n290 = stacked-sequence {
              frame #0 {
                n291 = Wait (ms)(milliseconds to wait=u32 1500) -> ()  [unwired: 1 out]
              }
              frame #1 {
                n292 = local read "Set Temp"() -> (w375:dbl)
                n293 = Number To Fractional String(number=w375, precision (6)=i16 2) -> (F-format string=w378:string)  [unwired: 2 in]
                n294 = Concatenate Strings("ST;" ("Command"), w378) -> (w377:string)
                n295 = local write "Due Write"(w377) -> ()
              }
              frame #2 {
                n296 = Wait (ms)(milliseconds to wait=u32 1500) -> ()  [unwired: 1 out]
              }
              frame #3 {
                n297 = local write "Due Write"("HE;1" ("Command")) -> ()
              }
              frame #4 {
                n298 = Wait (ms)(milliseconds to wait=u32 1500) -> ()  [unwired: 1 out]
              }
              frame #5 {
                n299 = stacked-sequence {
                  frame #0 {
                    n300 = Wait (ms)(milliseconds to wait=u32 1500) -> ()  [unwired: 1 out]
                  }
                  frame #1 {
                    n301 = local read "Set Temp"() -> (w384:dbl)
                    n302 = Number To Fractional String(number=w384, precision (6)=i16 2) -> (F-format string=w387:string)  [unwired: 2 in]
                    n303 = Concatenate Strings("ST;" ("Command"), w387) -> (w386:string)
                    n304 = local write "Due Write"(w386) -> ()
                  }
                  frame #2 {
                    n305 = Wait (ms)(milliseconds to wait=u32 1500) -> ()  [unwired: 1 out]
                  }
                  frame #3 {
                    n306 = local write "Due Write"("HE;1" ("Command")) -> ()
                  }
                  frame #4 {
                    n307 = Wait (ms)(milliseconds to wait=u32 1500) -> ()  [unwired: 1 out]
                  }
                }
              }
            }
          }
          frame False {
            n308 = stacked-sequence {
              frame #0 {
                n309 = Wait (ms)(milliseconds to wait=u32 1500) -> ()  [unwired: 1 out]
              }
              frame #1 {
                n310 = Concatenate Strings("ST;" ("Command"), "0" ("string")) -> (w394:string)
                n311 = local write "Due Write"(w394) -> ()
              }
              frame #2 {
                n312 = Wait (ms)(milliseconds to wait=u32 1500) -> ()  [unwired: 1 out]
              }
              frame #3 {
                n313 = local write "Due Write"("HE;0" ("Command")) -> ()
              }
              frame #4 {
                n314 = Wait (ms)(milliseconds to wait=u32 1500) -> ()  [unwired: 1 out]
              }
            }
          }
        }
      }
      event "Headen Service Button": Value Change {
        n315 = event-data() -> ()  [unwired: 1 in, 6 out]
        n316 = local read "Headen Service Button"() -> (w399:bool)
        n317 = case shown="True" w399 {
          frame False {
            n318 = property on="Password 3" class="Clust (strict)"("Visible"=FALSE) -> ()  [unwired: 2 in, 2 out]
            n319 = property on="Service Password Log" class="Str"("Visible"=FALSE) -> ()  [unwired: 2 in, 2 out]
          }
          frame True {
            n320 = property on="Password 3" class="Clust (strict)"("Visible"=TRUE) -> ()  [unwired: 2 in, 2 out]
            n321 = property on="Service Password Log" class="Str"("Visible"=TRUE) -> ()  [unwired: 2 in, 2 out]
          }
        }
      }
      event "Password 3.Service Password": Value Change {
